vi "GetOutputWaveform.vi"(8 "error in (no error)":errorcluster, 11 "FunctionGenerator in":refnum<class "FunctionGenerator.lvclass">) -> (0 "error out":errorcluster, 2 "OutputWaveform.lvclass":refnum<class "OutputWaveform.lvclass">, 3 "FunctionGenerator out":refnum<class "FunctionGenerator.lvclass">)   [LabVIEW 2020, in "FunctionGenerator.lvclass"]
uses:
  FunctionGenerator.lvclass
  OutputWaveform/OutputWaveform.lvclass
  FunctionGenerator.lvclass/FunctionGenerator.ctl
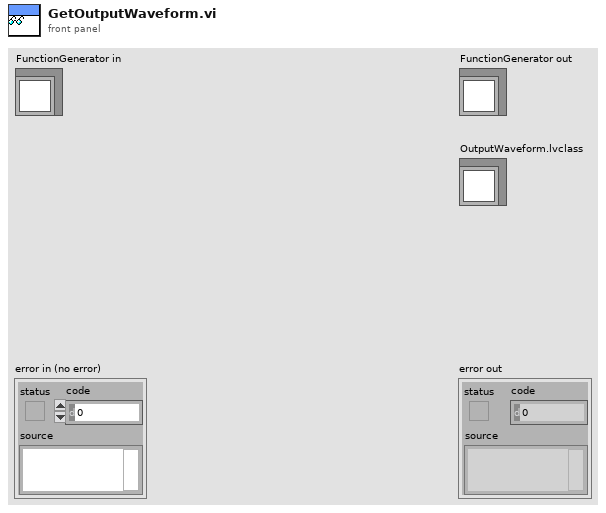
[diagram p1: front panel]
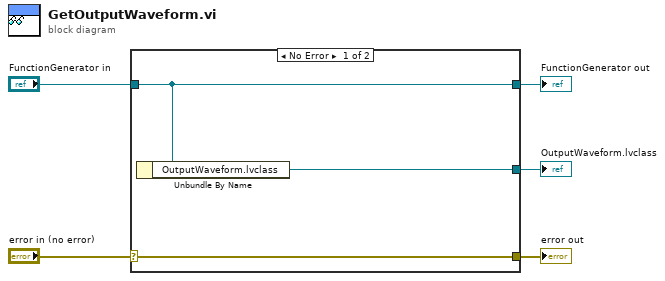
[diagram p0: block diagram]
diagram:
  n1 = case shown="No Error" "error in (no error)" {
    selector: "error in (no error)" -> [w8 w9]
    tunnel: [w8 w9] -> w4
    tunnel: [w7 w10] -> w2
    tunnel: "FunctionGenerator in" -> [w7 w10]
    tunnel: [w6 _] -> w1
    frame No Error {
      n2 = Unbundle By Name(w7) -> ("OutputWaveform.lvclass"=w6:refnum<class "OutputWaveform.lvclass">)
    }
    frame Error {
    }
  }
  "error out" <- w4
  "FunctionGenerator out" <- w2
  "OutputWaveform.lvclass" <- w1
